vi "Example 0.vi"   [LabVIEW 2014, in "Baskett_Jaques_5th_LEGORobotics_11-29-16.lvrbt"]
uses:
  Baskett_Jaques_5th_LEGORobotics_11-29-16.lvrbt
  <vilib>/NXT/Dual Mode Library/Display/drawText.vi
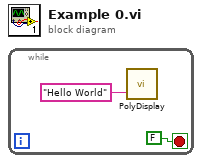
[diagram p0: block diagram]
diagram:
  n1 = while {
    stop <- FALSE stop-if-true
    n2 = call-poly <vilib>:"PolyDisplay.vi"("Text"="Hello World") -> ()  [unwired: 3 in, 1 out]
  }
